vi "Latihan 9 (Traffic Light).vi"() -> ()   [LabVIEW 2021]
panel:
  out "Slide 5":dbl(slide) scale=0.0..10.0
  out "Slide":dbl(slide)
  out "Slide 3":dbl(slide)=10.0
  out "Slide 2":dbl(slide) scale=0.0..10.0
  in  "stop":bool
  in  "Lampu 4":enum32{"Page 1"}(tab)
  out "Merah 4":bool
  out "Hijau 4":bool
  out "Kuning 4":bool
  in  "Lampu 3":enum32{"Page 1"}(tab)
  out "Merah 3":bool
  out "Hijau 3":bool
  out "Kuning 3":bool
  in  "Lampu 2":enum32{"Page 1"}(tab)
  out "Hijau 2":bool
  out "Merah 2":bool
  out "Kuning 2":bool
  in  "Lampu 1":enum32{"Page 1"}(tab)
  out "Hijau 1":bool
  out "Merah 1":bool
  out "Kuning 1":bool
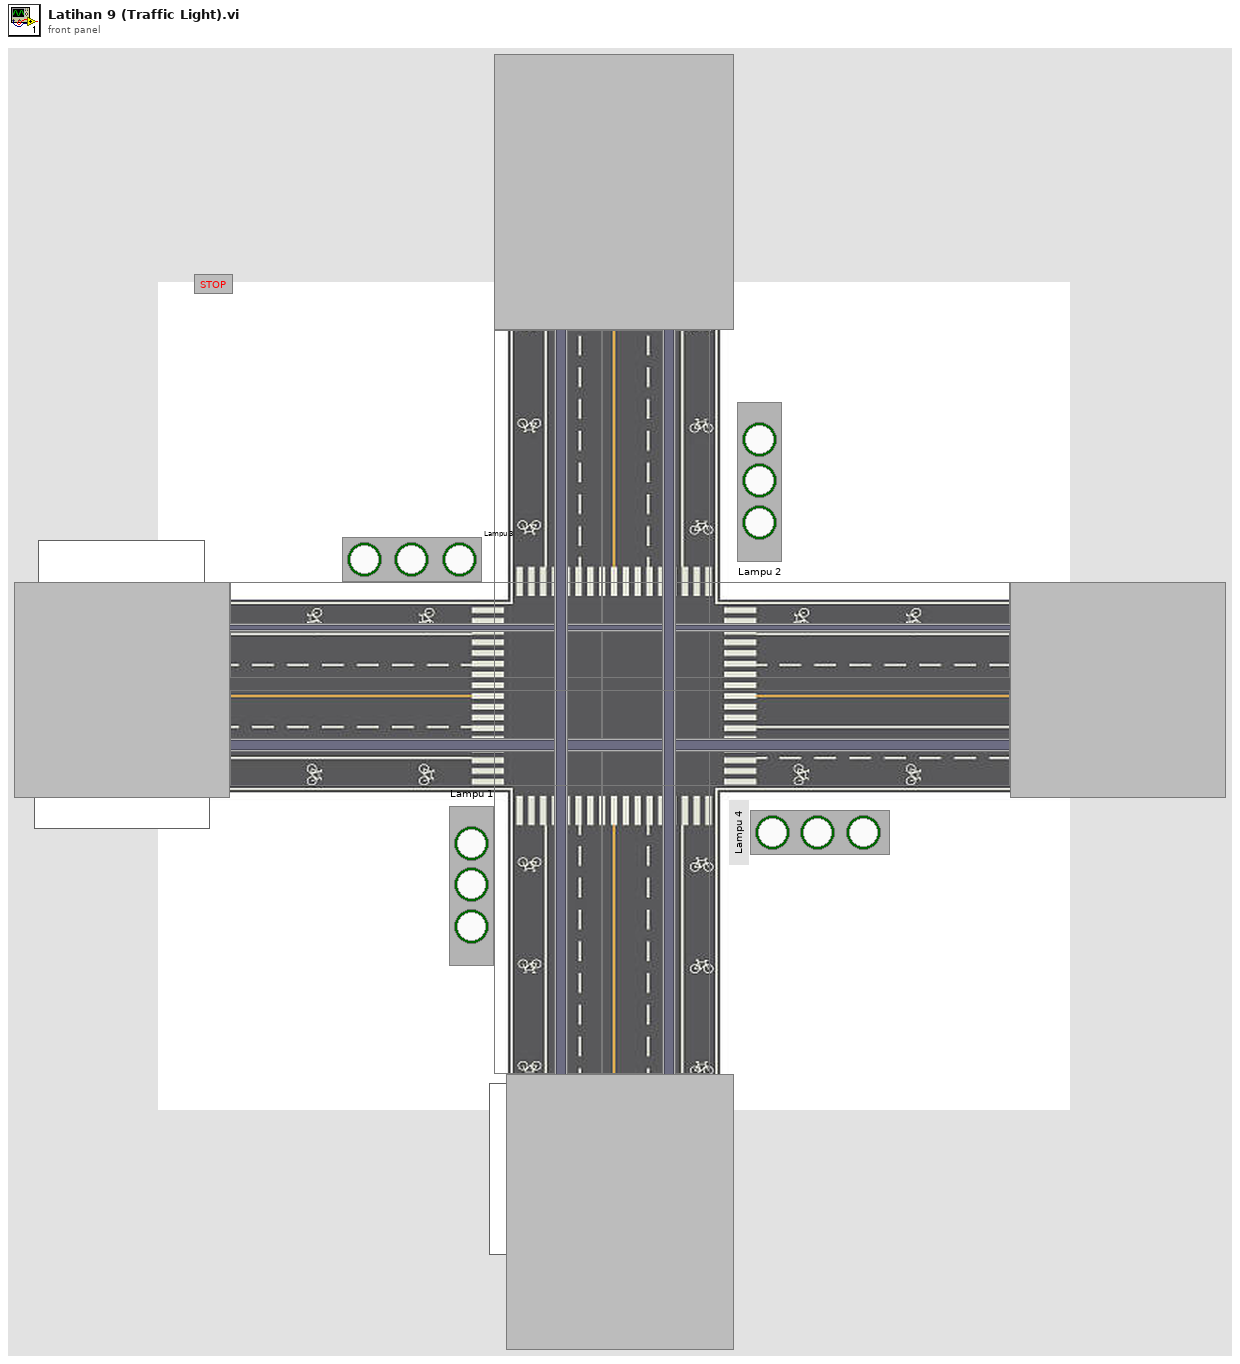
[diagram p1: front panel]
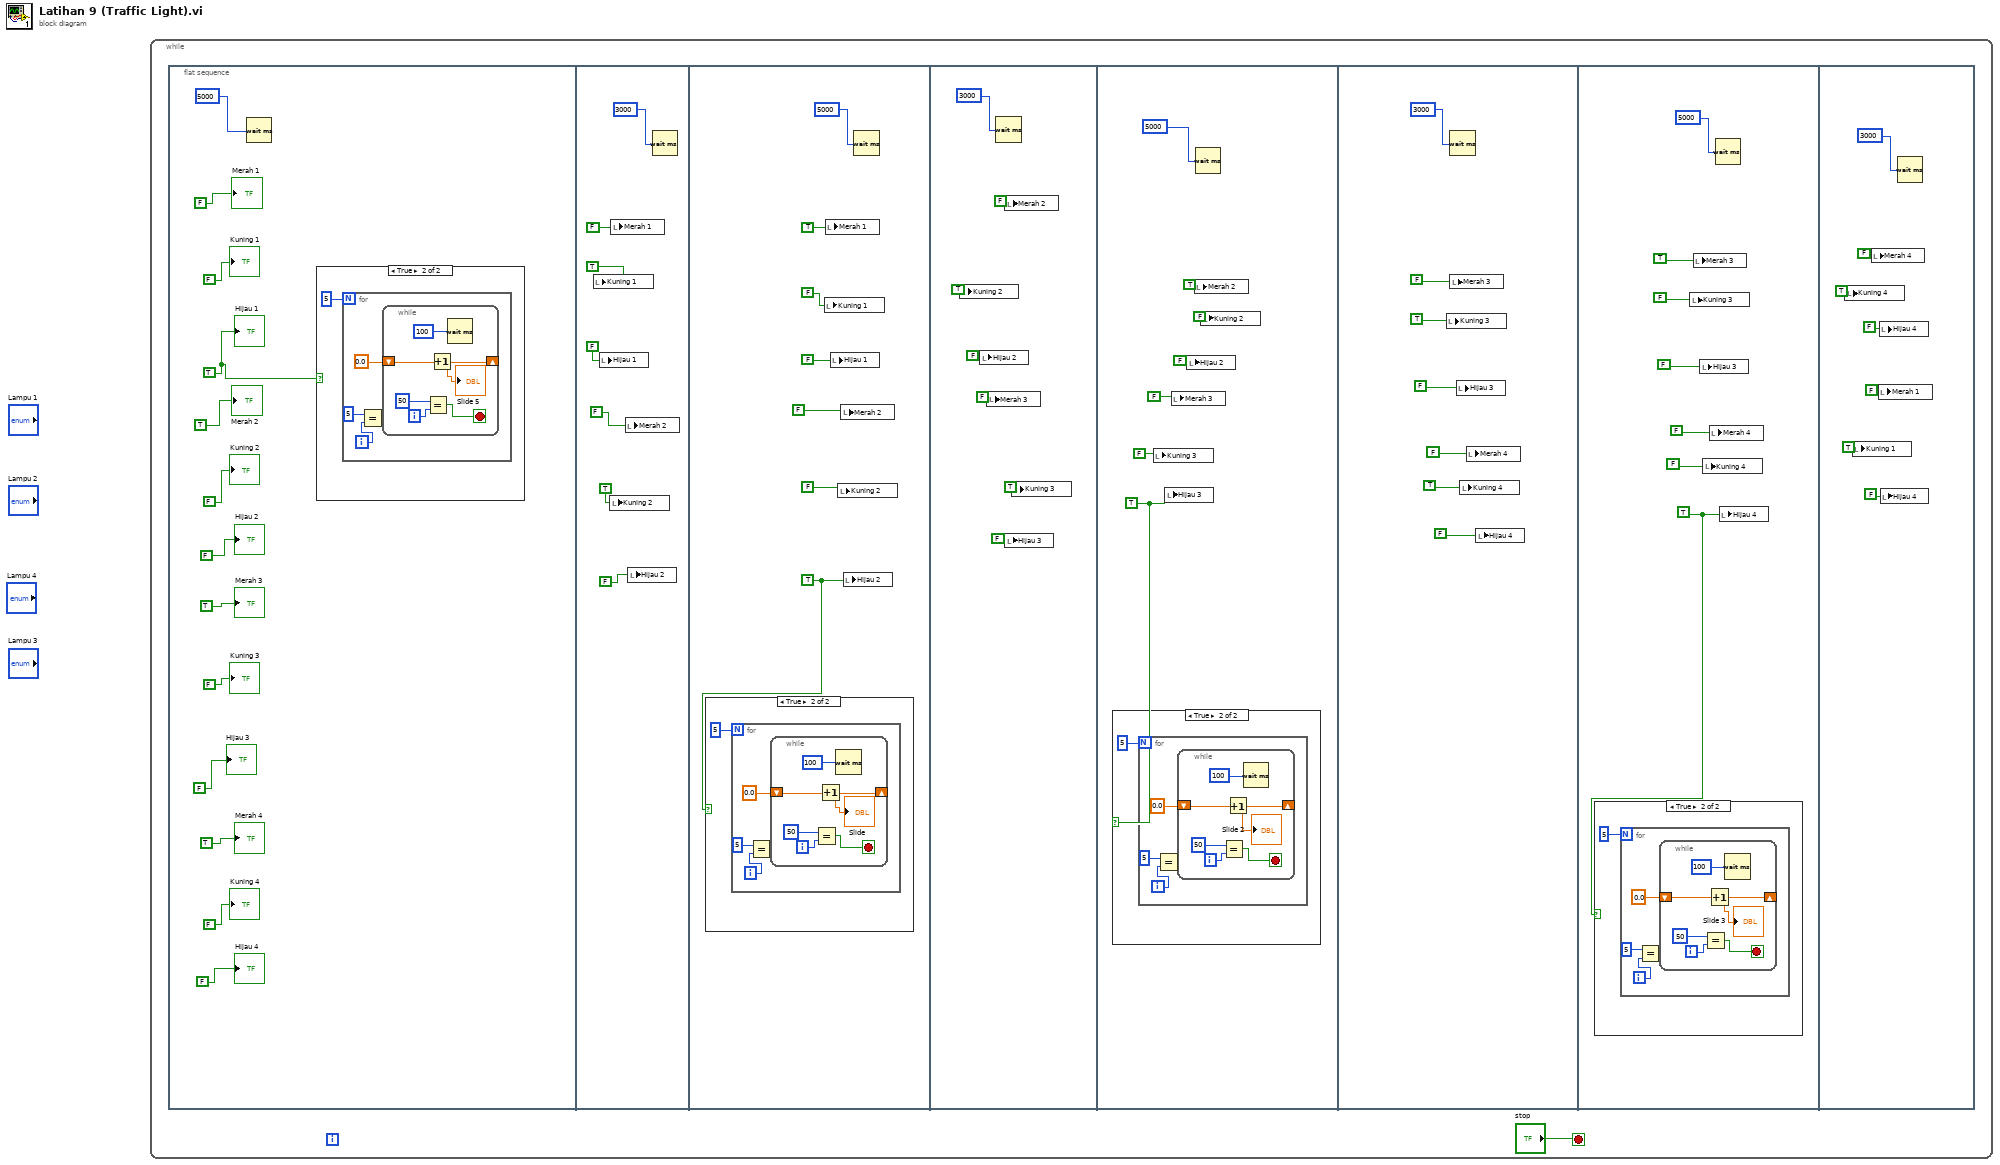
[diagram p0: block diagram]
diagram:
  n1 = while {
    stop <- "stop" stop-if-true
    n2 = flat-sequence {
      frame #0 {
        w2 = TRUE
        n3 = Wait (ms)(milliseconds to wait=u32 5000) -> ()  [unwired: 1 out]
        n4 = case shown="True" w2 {
          frame False {
          }
          frame True {
            n5 = for {
              N: 5 -> [_]
              i -> [w17]
              n6 = Equal?(x=5, y=w17) -> ()  [unwired: 1 out]
              n7 = while {
                shift-right: [w19] -> _
                shift-left: 0.0 -> [w21]
                i -> [w24]
                stop <- w22 stop-if-true
                n8 = Equal?(x=50, y=w24) -> (x = y?=w22:bool)
                n9 = Increment(x=w21) -> (x+1=w19:dbl)
                "Slide 5" <- w19
                n10 = Wait (ms)(milliseconds to wait=u32 100) -> ()  [unwired: 1 out]
              }
            }
          }
        }
        "Merah 1" <- FALSE
        "Hijau 1" <- w2
        "Kuning 1" <- FALSE
        "Hijau 2" <- FALSE
        "Merah 2" <- TRUE
        "Kuning 2" <- FALSE
        "Merah 3" <- TRUE
        "Kuning 3" <- FALSE
        "Merah 4" <- TRUE
        "Kuning 4" <- FALSE
        "Hijau 3" <- FALSE
        "Hijau 4" <- FALSE
      }
      frame #1 {
        n11 = local write "Kuning 1"(TRUE) -> ()
        n12 = local write "Hijau 1"(FALSE) -> ()
        n13 = local write "Kuning 2"(TRUE) -> ()
        n14 = local write "Merah 1"(FALSE) -> ()
        n15 = local write "Merah 2"(FALSE) -> ()
        n16 = local write "Hijau 2"(FALSE) -> ()
        n17 = Wait (ms)(milliseconds to wait=u32 3000) -> ()  [unwired: 1 out]
      }
      frame #2 {
        w32 = TRUE
        n18 = case shown="True" w32 {
          frame False {
          }
          frame True {
            n19 = for {
              N: 5 -> [_]
              i -> [w41]
              n20 = Equal?(x=5, y=w41) -> ()  [unwired: 1 out]
              n21 = while {
                shift-right: [w43] -> _
                shift-left: 0.0 -> [w45]
                i -> [w48]
                stop <- w46 stop-if-true
                n22 = Equal?(x=50, y=w48) -> (x = y?=w46:bool)
                n23 = Increment(x=w45) -> (x+1=w43:dbl)
                "Slide" <- w43
                n24 = Wait (ms)(milliseconds to wait=u32 100) -> ()  [unwired: 1 out]
              }
            }
          }
        }
        n25 = local write "Kuning 1"(FALSE) -> ()
        n26 = local write "Merah 1"(TRUE) -> ()
        n27 = local write "Hijau 1"(FALSE) -> ()
        n28 = local write "Kuning 2"(FALSE) -> ()
        n29 = local write "Merah 2"(FALSE) -> ()
        n30 = local write "Hijau 2"(w32) -> ()
        n31 = Wait (ms)(milliseconds to wait=u32 5000) -> ()  [unwired: 1 out]
      }
      frame #3 {
        n32 = local write "Kuning 2"(TRUE) -> ()
        n33 = local write "Hijau 2"(FALSE) -> ()
        n34 = local write "Merah 3"(FALSE) -> ()
        n35 = Wait (ms)(milliseconds to wait=u32 3000) -> ()  [unwired: 1 out]
        n36 = local write "Merah 2"(FALSE) -> ()
        n37 = local write "Hijau 3"(FALSE) -> ()
        n38 = local write "Kuning 3"(TRUE) -> ()
      }
      frame #4 {
        w56 = TRUE
        n39 = case shown="True" w56 {
          frame False {
          }
          frame True {
            n40 = for {
              N: 5 -> [_]
              i -> [w65]
              n41 = Equal?(x=5, y=w65) -> ()  [unwired: 1 out]
              n42 = while {
                shift-right: [w69] -> _
                shift-left: 0.0 -> [w68]
                i -> [w72]
                stop <- w70 stop-if-true
                n43 = Equal?(x=50, y=w72) -> (x = y?=w70:bool)
                n44 = Increment(x=w68) -> (x+1=w69:dbl)
                "Slide 2" <- w69
                n45 = Wait (ms)(milliseconds to wait=u32 100) -> ()  [unwired: 1 out]
              }
            }
          }
        }
        n46 = local write "Kuning 3"(FALSE) -> ()
        n47 = local write "Hijau 3"(w56) -> ()
        n48 = local write "Merah 3"(FALSE) -> ()
        n49 = local write "Hijau 2"(FALSE) -> ()
        n50 = local write "Merah 2"(TRUE) -> ()
        n51 = Wait (ms)(milliseconds to wait=u32 5000) -> ()  [unwired: 1 out]
        n52 = local write "Kuning 2"(FALSE) -> ()
      }
      frame #5 {
        n53 = local write "Kuning 3"(TRUE) -> ()
        n54 = Wait (ms)(milliseconds to wait=u32 3000) -> ()  [unwired: 1 out]
        n55 = local write "Merah 3"(FALSE) -> ()
        n56 = local write "Hijau 3"(FALSE) -> ()
        n57 = local write "Kuning 4"(TRUE) -> ()
        n58 = local write "Merah 4"(FALSE) -> ()
        n59 = local write "Hijau 4"(FALSE) -> ()
      }
      frame #6 {
        w80 = TRUE
        n60 = case shown="True" w80 {
          frame False {
          }
          frame True {
            n61 = for {
              N: 5 -> [_]
              i -> [w89]
              n62 = Equal?(x=5, y=w89) -> ()  [unwired: 1 out]
              n63 = while {
                shift-right: [w91] -> _
                shift-left: 0.0 -> [w93]
                i -> [w96]
                stop <- w94 stop-if-true
                n64 = Equal?(x=50, y=w96) -> (x = y?=w94:bool)
                n65 = Increment(x=w93) -> (x+1=w91:dbl)
                "Slide 3" <- w91
                n66 = Wait (ms)(milliseconds to wait=u32 100) -> ()  [unwired: 1 out]
              }
            }
          }
        }
        n67 = local write "Kuning 3"(FALSE) -> ()
        n68 = local write "Merah 3"(TRUE) -> ()
        n69 = local write "Hijau 3"(FALSE) -> ()
        n70 = local write "Kuning 4"(FALSE) -> ()
        n71 = local write "Merah 4"(FALSE) -> ()
        n72 = Wait (ms)(milliseconds to wait=u32 5000) -> ()  [unwired: 1 out]
        n73 = local write "Hijau 4"(w80) -> ()
      }
      frame #7 {
        n74 = local write "Kuning 4"(TRUE) -> ()
        n75 = local write "Kuning 1"(TRUE) -> ()
        n76 = local write "Merah 4"(FALSE) -> ()
        n77 = local write "Merah 1"(FALSE) -> ()
        n78 = local write "Hijau 4"(FALSE) -> ()
        n79 = local write "Hijau 4"(FALSE) -> ()
        n80 = Wait (ms)(milliseconds to wait=u32 3000) -> ()  [unwired: 1 out]
      }
    }
  }
